vi "FFT_averaging.vi"(0 "dt":dbl, 1 "chirp end":dbl, 2 "frame":i32, 3 "current frequency":dbl, 5 "3d waveform array":dbl[][][](array[numeric]), 8 "reset frame average":bool, 10 "all frames?":bool) -> (9 "BG waveform":waveform(dbl), 11 "Mol waveform":waveform(dbl), 12 "averages compl":i32, 13 "cor waveform":waveform(dbl), 14 "BG spectrum":T1, 16 "Mol spectrum":T1(graph), 18 "cor spectrum":T1(graph))   [LabVIEW 2011]
uses:
  global.vi
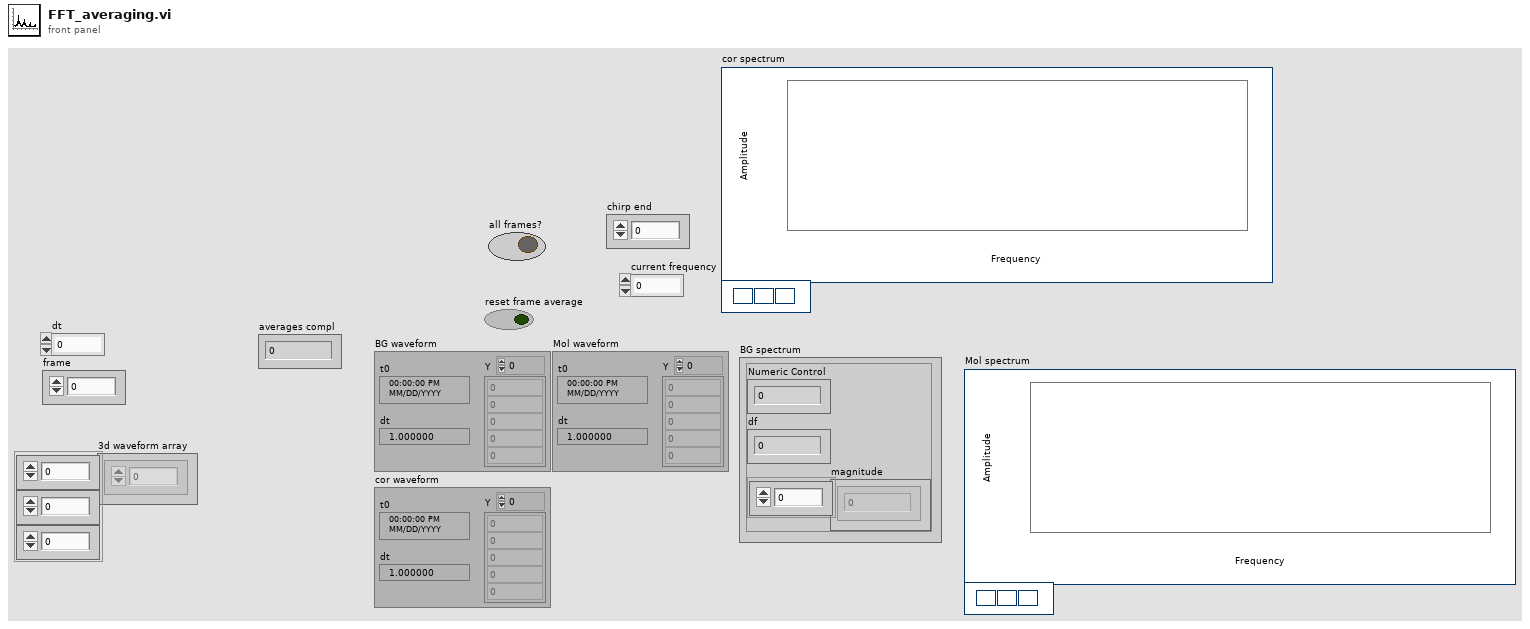
[diagram p1: front panel]
types:
  T1 = cluster{"Numeric Control":dbl, "df":dbl, "magnitude":dbl[]}
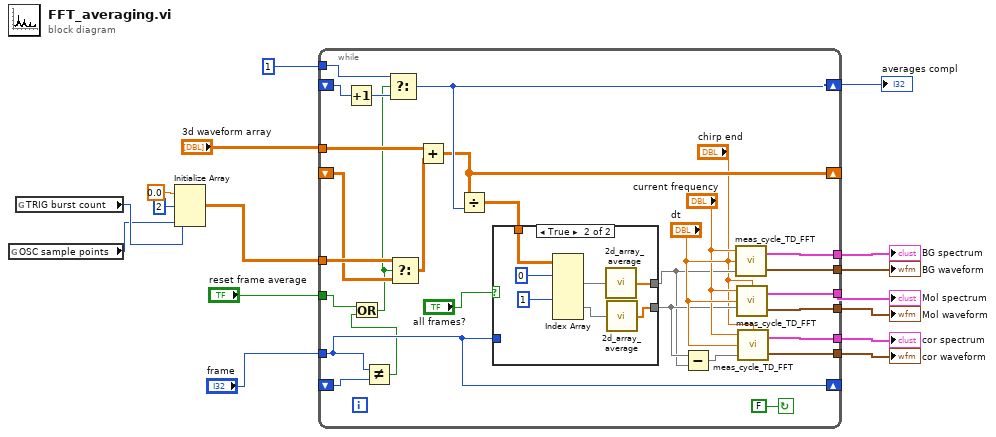
[diagram p0: block diagram]
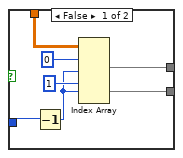
[diagram p2: hidden frame]
diagram:
  n1 = global read "global.vi" "OSC sample points"() -> (w11:i32)
  n2 = global read "global.vi" "TRIG burst count"() -> (w15:i32)
  n3 = Initialize Array(0.0 ("element"), 2 ("dimension size"), w15, w11) -> (w13:dbl[][][])
  n4 = while {
    shift-right: [w34] -> _
    shift-left: _ -> [w43]
    tunnel: w13 -> [w44]
    tunnel: "reset frame average" -> [w19]
    tunnel: "3d waveform array" -> [w41]
    shift-right: [w35] -> w9
    shift-left: _ -> [w40]
    tunnel: 1 -> [w38]
    tunnel: [w36] -> w8
    tunnel: [w37] -> w7
    tunnel: [w26] -> w5
    tunnel: [w25] -> w4
    tunnel: [w24] -> w3
    tunnel: [w23] -> w2
    tunnel: "frame" -> [w20]
    shift-right: [w20] -> _
    shift-left: _ -> [w21]
    stop <- FALSE continue-if-true
    n5 = Increment(x=w40) -> (x+1=w39:i32)
    n6 = Not Equal?(x=w20, y=w21) -> (x != y?=w17:bool)
    n7 = Or(x=w19, y=w17) -> (x .or. y?=w18:bool)
    n8 = Select(t=w38, s=w18, f=w39) -> (s? t:f=w35:i32)
    n9 = Select(t=w44, s=w18, f=w43) -> (s? t:f=w42:dbl[][][])
    n10 = Add(x=w41, y=w42) -> (x+y=w34:dbl[][][])
    n11 = Divide(x=w34, y=w35) -> (x/y=w33:dbl[][][])
    n12 = case shown="True" "all frames?" {
      tunnel: [w49 w54] -> w29
      tunnel: w20 -> [w48 _]
      tunnel: [w47 w56] -> w28
      tunnel: w33 -> [w46 w57]
      frame False {
        n13 = Decrement(x=w48) -> (x-1=w50:i32)
        n14 = Index Array(array=w46, index (dim 0) #1=0 ("disabled index (page)"), index (dim 1) #1=w50, index (dim 0) #2=1 ("disabled index (page)"), index (dim 1) #2=w50) -> (element #1=w47:dbl[], element #2=w49:dbl[])  [unwired: 2 in]
      }
      frame True {
        n15 = Index Array(array=w57, index (dim 0) #1=0 ("disabled index (page)"), index (dim 0) #2=1 ("disabled index (page)")) -> (element #1=w53:dbl[][], element #2=w55:dbl[][])  [unwired: 4 in]
        n16 = call "2d_array_average.vi"("2D array"=w53) -> ("array average"=w56:dbl[])  [unwired: 4 in]
        n17 = call "2d_array_average.vi"("2D array"=w55) -> ("array average"=w54:dbl[])  [unwired: 4 in]
      }
    }
    n18 = Subtract(x=w29, y=w28) -> (x-y=w27:dbl[])
    n19 = call "meas_cycle_TD_FFT.vi"("chirp end"="chirp end", "time domain array"=w28, "dt"="dt", "current frequency"="current frequency") -> ("output time domain signal"=w25:waveform(dbl), "output spectrum"=w36:T1)
    n20 = call "meas_cycle_TD_FFT.vi"("chirp end"="chirp end", "time domain array"=w29, "dt"="dt", "current frequency"="current frequency") -> ("output time domain signal"=w24:waveform(dbl), "output spectrum"=w37:T1)
    n21 = call "meas_cycle_TD_FFT.vi"("chirp end"="chirp end", "time domain array"=w27, "dt"="dt", "current frequency"="current frequency") -> ("output time domain signal"=w23:waveform(dbl), "output spectrum"=w26:T1)
  }
  "averages compl" <- w9
  "Mol spectrum" <- w7
  "cor spectrum" <- w5
  "BG spectrum" <- w8
  "BG waveform" <- w4
  "Mol waveform" <- w3
  "cor waveform" <- w2
